vi "SHAPE_displaySolution.vi"(7 "Class Label":refnum<vi>, 8 "Stop Notifier In":refnum<notifier>, 9 "Control Refs":T1, 10 "Solution notifier":refnum<notifier>, 11 "BandGlobalOpt.lvclass":refnum<class "Shapelets Search GA.lvclass">) -> ()   [LabVIEW 2016, in "Shapelets Search (GA).lvlib" / "Shapelets Search GA.lvclass"]
uses:
  Shapelets Search GA.lvclass
  5. Features Optimization/_Optimal Frequency Bands Search/GA_core/GA_tSolution progress.ctl
  Shapelets Search GA.lvclass/Shapelets Search GA.ctl
  5. Features Optimization/_Optimal Frequency Bands Search/GA_core/GeneticAlgorithm.lvlib
panel:
  out "ShapeletForm":cluster{i32[], dbl[]}[](array[cluster])
  # "This VI is a part of BCI Design library, http://www.ru-bci.org \nCopyright © 2020, Sotnikov Peter, All rights reserved. License: CC BY-NC 4.0"
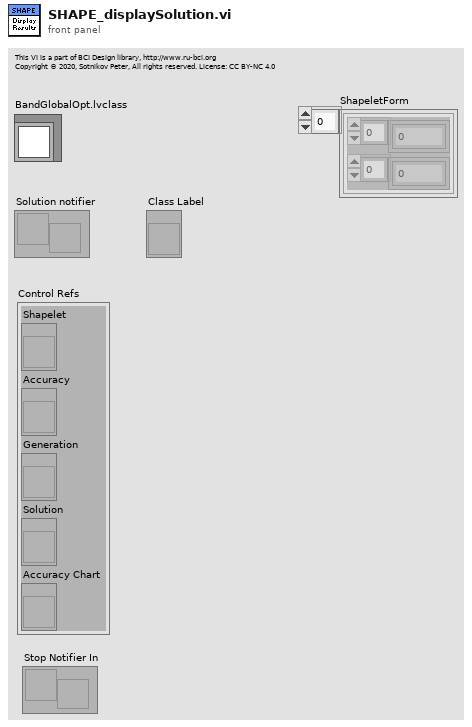
[diagram p1: front panel]
types:
  T1 = cluster{"Shapelet":refnum<vi>, "Accuracy":refnum<vi>, "Generation":refnum<vi>, "Solution":refnum<vi>, "Accuracy Chart":refnum<vi>}
  T2 = typedef "Optimal Frequency Bands Search.lvlib/GeneticAlgorithm.lvlib/GA_tSolution progress.ctl" = cluster{"Solution":i32[], "Fitness":dbl, "Mutation rate":dbl, "Generation":i32}
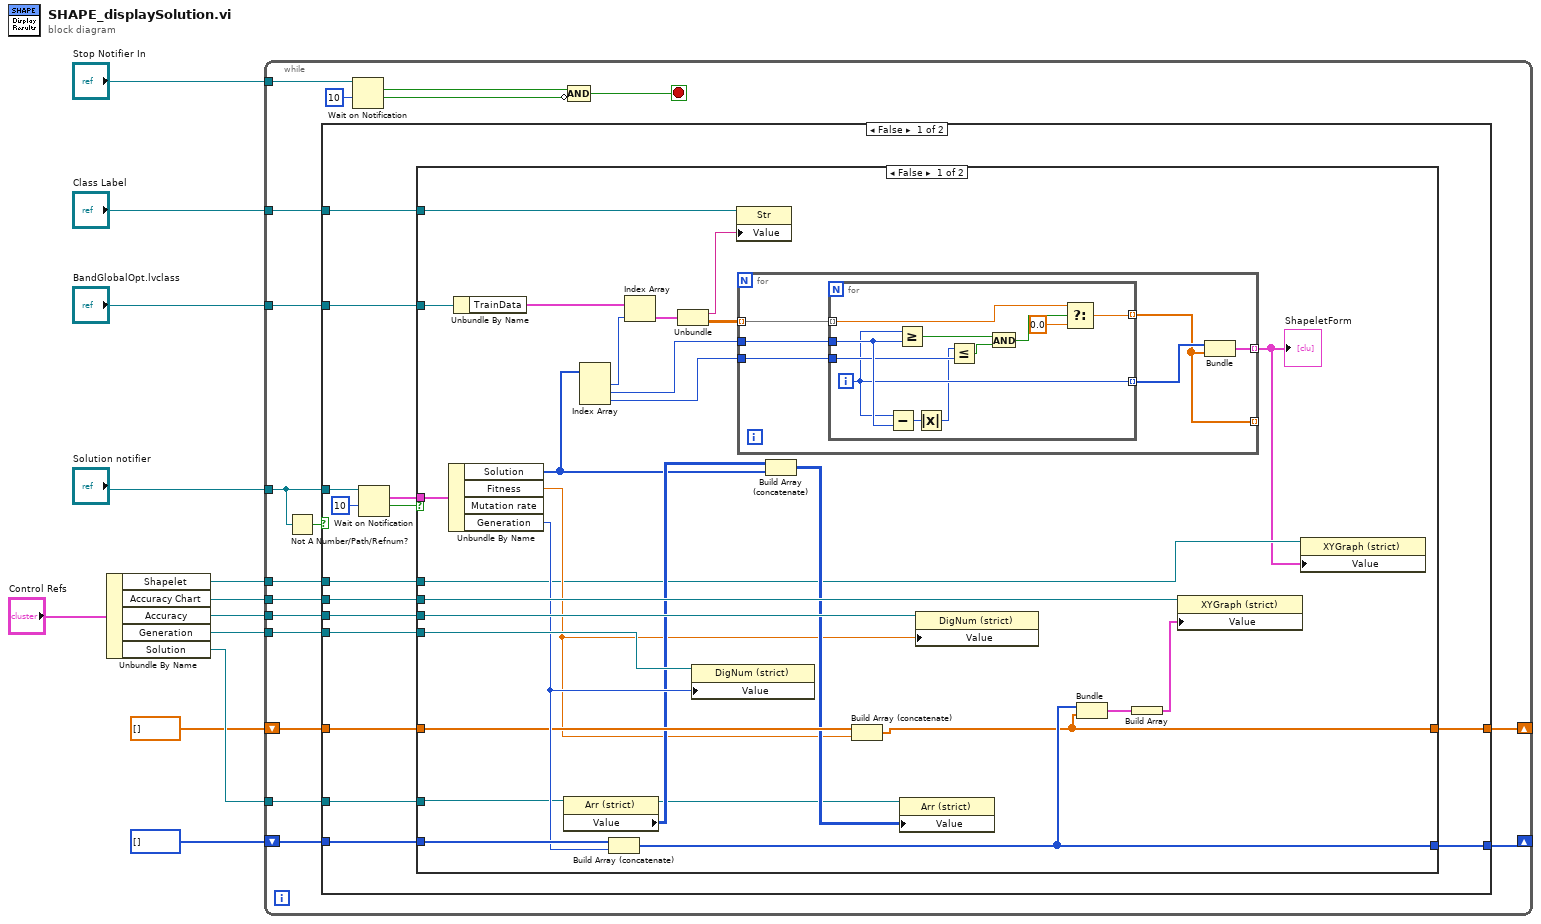
[diagram p0: block diagram]
diagram:
  n1 = Unbundle By Name("Control Refs") -> ("Shapelet"=w2:refnum<vi>, "Accuracy Chart"=w11:refnum<vi>, "Accuracy"=w10:refnum<vi>, "Generation"=w9:refnum<vi>, "Solution"=w8:refnum<vi>)
  n2 = while {
    tunnel: "Solution notifier" -> [w29]
    tunnel: "Stop Notifier In" -> [w28]
    tunnel: w11 -> [w23]
    tunnel: w10 -> [w22]
    tunnel: w9 -> [w21]
    tunnel: w8 -> [w20]
    shift-right: [w18] -> _
    shift-left: i32[] [] -> [w19]
    shift-right: [w16] -> _
    shift-left: dbl[] [] -> [w17]
    tunnel: "BandGlobalOpt.lvclass" -> [w15]
    tunnel: w2 -> [w14]
    tunnel: "Class Label" -> [w13]
    stop <- w24 stop-if-true
    n3 = Not A Number/Path/Refnum?(number/path/refnum=w29) -> (NaN/Path/Refnum?=w30:bool)
    n4 = case shown="False" w30 {
      tunnel: w29 -> [w45 _]
      tunnel: w23 -> [w41 _]
      tunnel: w22 -> [w40 _]
      tunnel: w21 -> [w39 _]
      tunnel: w20 -> [w38 _]
      tunnel: w19 -> [w37 w94]
      tunnel: [w36 w94] -> w18
      tunnel: w17 -> [w35 w93]
      tunnel: [w34 w93] -> w16
      tunnel: w15 -> [w33 _]
      tunnel: w14 -> [w32 _]
      tunnel: w13 -> [w31 _]
      frame False {
        n5 = Wait on Notification(notifier=w45, timeout in ms (-1)=10) -> (notification=w43:T2, timed out?=w44:bool)  [unwired: 2 in, 2 out]
        n6 = case shown="False" w44 {
          tunnel: w43 -> [w73 _]
          tunnel: w41 -> [w72 _]
          tunnel: w40 -> [w71 _]
          tunnel: w39 -> [w70 _]
          tunnel: w38 -> [w63 _]
          tunnel: w37 -> [w69 w92]
          tunnel: [w66 w92] -> w36
          tunnel: w35 -> [w67 w91]
          tunnel: [w65 w91] -> w34
          tunnel: w33 -> [w56 _]
          tunnel: w32 -> [w49 _]
          tunnel: w31 -> [w47 _]
          frame False {
            n7 = Unbundle By Name(w73) -> ("Solution"=w54:i32[], "Fitness"=w59:dbl, "Generation"=w68:i32)  [unwired: 1 out]
            n8 = Unbundle By Name(w56) -> ("TrainData"=w55:cluster{"ClassLabel":string, "Trial":dbl[][]}[])
            n9 = property class="Arr (strict)"(reference=w63) -> (reference out=w60:refnum<vi>, "Value"=w62:i32[][])  [unwired: 1 in, 1 out]
            n10 = Index Array(array=w54) -> (element #1=w53:i32, element #2=w52:i32, element #3=w51:i32)  [unwired: 3 in]
            n11 = Build Array (concatenate)(w69, w68) -> (w66:i32[])
            n12 = Index Array(array=w55, index=w53) -> (element=w58:cluster{"ClassLabel":string, "Trial":dbl[][]})
            n13 = Unbundle(w58) -> ("ClassLabel"=w46:string, "Trial"=w57:dbl[][])
            n14 = property class="DigNum (strict)"(reference=w70, "Value"=w68) -> ()  [unwired: 1 in, 2 out]
            n15 = property class="Str"(reference=w47, "Value"=w46) -> ()  [unwired: 1 in, 2 out]
            n16 = for {
              tunnel: w57 -> [w74] mode=indexing
              tunnel: w52 -> [w79]
              tunnel: w51 -> [w78]
              tunnel: [w76] -> w48 mode=indexing
              tunnel: [w75] -> _ mode=indexing
              n17 = for {
                tunnel: w74 -> [w81] mode=indexing
                tunnel: w79 -> [w90]
                tunnel: w78 -> [w89]
                tunnel: [w80] -> w75 mode=indexing
                tunnel: [w84] -> w77 mode=indexing
                i -> [w84]
                n18 = Subtract(x=w84, y=w90) -> (x-y=w83:i32)
                n19 = Greater Or Equal?(x=w84, y=w90) -> (x >= y?=w88:bool)
                n20 = Absolute Value(x=w83) -> (abs(x)=w82:i32)
                n21 = Less Or Equal?(x=w82, y=w89) -> (x <= y?=w87:bool)
                n22 = And(x=w88, y=w87) -> (x .and. y?=w86:bool)
                n23 = Select(t=w81, s=w86, f=0.0) -> (s? t:f=w80:dbl)
              }
              n24 = Bundle(w77, w75) -> (w76:cluster{i32[], dbl[]})  [unwired: 1 in]
            }
            "ShapeletForm" <- w48
            n25 = Build Array (concatenate)(w62, w54) -> (w61:i32[][])
            n26 = Build Array (concatenate)(w67, w59) -> (w65:dbl[])
            n27 = property class="Arr (strict)"(reference=w60, "Value"=w61) -> ()  [unwired: 1 in, 2 out]
            n28 = property class="DigNum (strict)"(reference=w71, "Value"=w59) -> ()  [unwired: 1 in, 2 out]
            n29 = Bundle(w66, w65) -> (w64:cluster{i32[], dbl[]})  [unwired: 1 in]
            n30 = Build Array(w64) -> (w50:cluster{i32[], dbl[]}[])
            n31 = property class="XYGraph (strict)"(reference=w72, "Value"=w50) -> ()  [unwired: 1 in, 2 out]
            n32 = property class="XYGraph (strict)"(reference=w49, "Value"=w48) -> ()  [unwired: 1 in, 2 out]
          }
          frame True {
          }
        }
      }
      frame True {
      }
    }
    n33 = Wait on Notification(notifier=w28, timeout in ms (-1)=10) -> (notification=w26:bool, timed out?=w25:bool)  [unwired: 2 in, 2 out]
    n34 = Compound Arithmetic op=AND(w26, invert w25) -> (w24:bool)
  }
